vi "Fpga-Reverse-U64.vi"(11 "Numeric in":u64) -> (3 "Numeric out":u64)   [LabVIEW 2017]
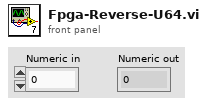
[diagram p1: front panel]
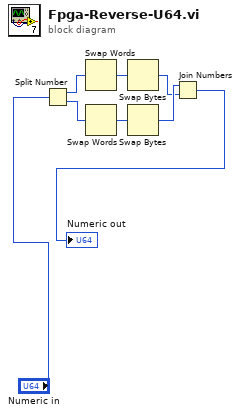
[diagram p0: block diagram]
diagram:
  n1 = Split Number(x="Numeric in") -> (hi(x)=w1:u32, lo(x)=w2:u32)
  n2 = Swap Words(1:w1) -> (0:w4:u32)
  n3 = Swap Words(1:w2) -> (0:w3:u32)
  n4 = Swap Bytes(anything=w4) -> (byte swapped=w5:u32)
  n5 = Swap Bytes(anything=w3) -> (byte swapped=w6:u32)
  n6 = Join Numbers(hi=w6, lo=w5) -> ((hi.lo)=→"Numeric out":u64)
